vi "DP-Plot IO Functions.vi"(1 "Plot refnum":refnum<vi>, 2 "Legend":refnum<vi>, 7 "Vals":dbl[](array[numeric]), 9 "Names in":string[](array[string]), 11 "error in":errorcluster, 12 "Value":cluster{"I-O Plot":dbl[], "I-O Plot":dbl[]}[](array[cluster]), 13 "noise":cluster{"I-O Plot":dbl[], "I-O Plot":dbl[]}[](array[cluster])) -> (10 "Names out":string[](array[string]), 15 "error out":errorcluster)   [LabVIEW 2020]
uses:
  epl-vi-lib/Utility VIs/Controls/KLegend/KLegend.xctl
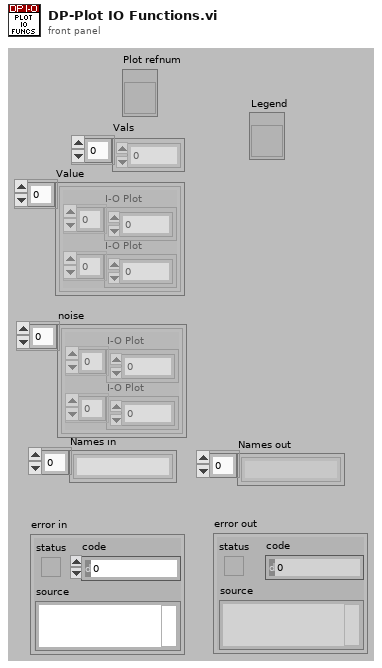
[diagram p1: front panel]
types:
  T1 = enum16{"User", "Prism", "Kelly", "Dark2", "Sequential", "Hue"}
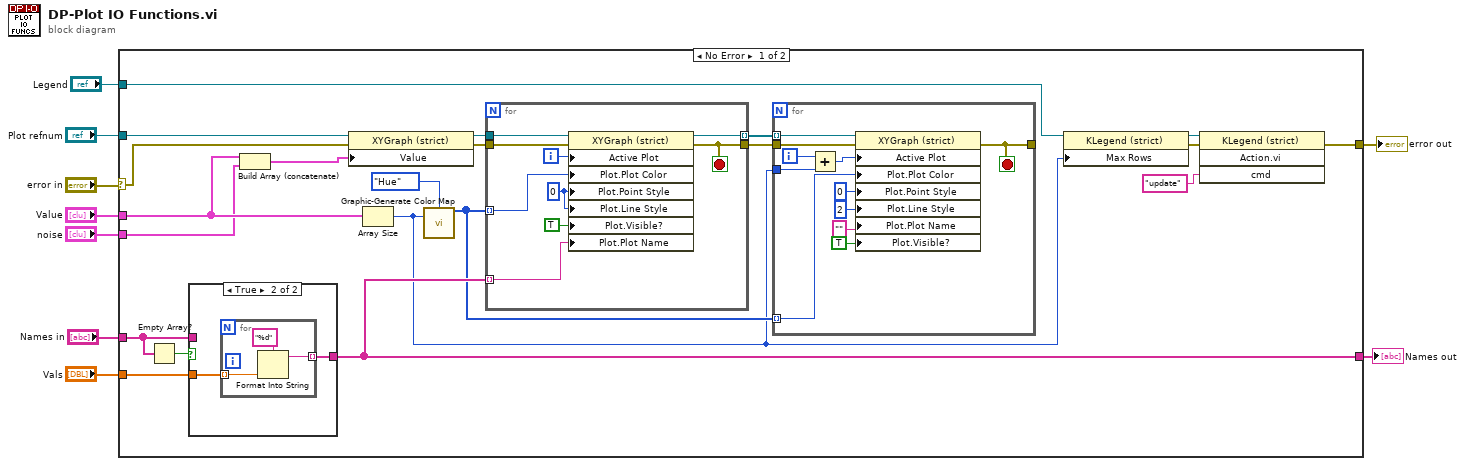
[diagram p0: block diagram]
diagram:
  n1 = case shown="No Error" "error in" {
    selector: "error in" -> [w28 w57]
    tunnel: "Vals" -> [w26 _]
    tunnel: "Plot refnum" -> [w30 _]
    tunnel: [w23 w57] -> w7
    tunnel: "Value" -> [w25 _]
    tunnel: "Legend" -> [w22 _]
    tunnel: [w20 _] -> w3
    tunnel: "Names in" -> [w19 _]
    tunnel: "noise" -> [w16 _]
    frame No Error {
      n2 = Empty Array?(array=w19) -> (empty?=w18:bool)
      n3 = case shown="True" w18 {
        tunnel: w26 -> [_ w33]
        tunnel: [w31 w32] -> w20
        tunnel: w19 -> [w31 _]
        frame False {
        }
        frame True {
          n4 = for {
            tunnel: w33 -> [w35] mode=indexing
            tunnel: [w34] -> w32 mode=indexing
            n5 = Format Into String(format string="%d", w35) -> (resulting string=w34:string)  [unwired: 2 in, 1 out]
          }
        }
      }
      n6 = Build Array (concatenate)(w25, w16) -> (w17:cluster{"I-O Plot":dbl[], "I-O Plot":dbl[]}[])
      n7 = property class="XYGraph (strict)"(reference=w30, error in=w28, "Value"=w17) -> (reference out=w29:refnum<vi>, error out=w27:errorcluster)
      n8 = Array Size(array=w25) -> (size(s)=w11:i32)
      n9 = call "Graphic-Generate Color Map.vi"("Map"=T1."Hue", "Size"=w11) -> ("Colors"=w13:u32[])  [unwired: 13 in]
      n10 = for {
        tunnel: w29 -> [w45]
        tunnel: w27 -> [w43]
        tunnel: [w42] -> w15
        tunnel: w20 -> [w41] mode=indexing
        tunnel: w13 -> [w40] mode=indexing
        tunnel: [w39] -> w14 mode=indexing
        i -> [w44]
        stop <- w42 stop-if-true
        w38 = u8 0 ("Plot.Point Style")
        n11 = property class="XYGraph (strict)"(reference=w45, error in=w43, "Active Plot"=w44, "Plot.Plot Color"=w40, "Plot.Point Style"=w38, "Plot.Line Style"=w38, "Plot.Visible?"=TRUE ("Plot.Visible"), "Plot.Plot Name"=w41) -> (reference out=w39:refnum<vi>, error out=w42:errorcluster)
      }
      n12 = for {
        tunnel: w14 -> [w56] mode=indexing
        tunnel: w15 -> [w54]
        tunnel: [w53] -> _
        tunnel: w13 -> [w52] mode=indexing
        tunnel: w11 -> [w48]
        i -> [w55]
        stop <- w53 stop-if-true
        n13 = Add(x=w55, y=w48) -> (x+y=w49:i32)
        n14 = property class="XYGraph (strict)"(reference=w56, error in=w54, "Active Plot"=w49, "Plot.Plot Color"=w52, "Plot.Point Style"=u8 0, "Plot.Line Style"=u8 2, "Plot.Plot Name"="", "Plot.Visible?"=TRUE ("Plot.Visible")) -> (error out=w53:errorcluster)  [unwired: 1 out]
      }
      n15 = property class="KLegend (strict)"(reference=w22, "Max Rows"=w11) -> (reference out=w12:refnum<vi>, error out=w10:errorcluster)  [unwired: 1 in]
      n16 = invoke class="KLegend (strict)" method="Action.vi"(reference=w12, error in=w10, "cmd"="update") -> (error out=w23:errorcluster)  [unwired: 1 in, 3 out]
    }
    frame Error {
    }
  }
  "error out" <- w7
  "Names out" <- w3
